vi "taskControllerExample.vi"() -> ()   [LabVIEW 2023]
uses:
  TaskController/TaskController.lvclass
  ITask/ITask.lvclass
panel:
  out "isRunning":bool
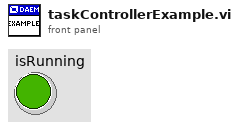
[diagram p1: front panel]
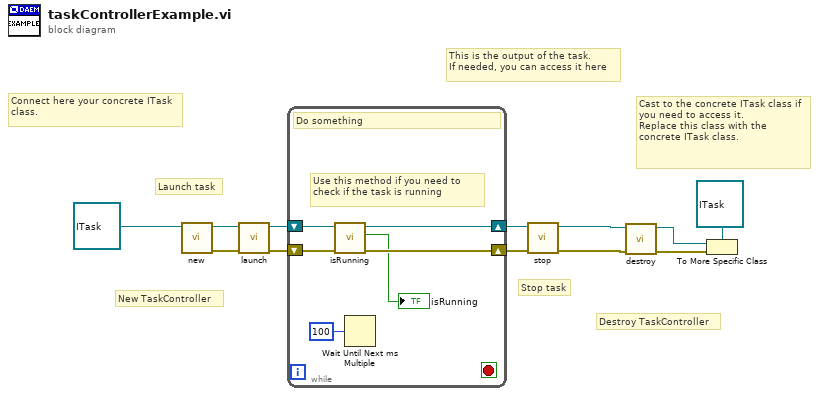
[diagram p0: block diagram]
diagram:
  # "Cast to the concrete ITask class if you need to access it.\nReplace this class with the concrete ITask class."
  # "This is the output of the task.\nIf needed, you can access it here"
  # "Connect here your concrete ITask class."
  # "Destroy TaskController"
  # "Stop task"
  # "Launch task"
  # "New TaskController"
  n1 = call "new.vi"("task"=refnum<class "ITask.lvclass"> refnum) -> ("error out"=w12:errorcluster, "TaskController out"=w11:refnum<class "TaskController.lvclass">)  [unwired: 9 in]
  n2 = call "launch.vi"("error in (no error)"=w12, "TaskController in"=w11) -> ("error out"=w10:errorcluster, "TaskController out"=w9:refnum<class "TaskController.lvclass">)  [unwired: 8 in]
  n3 = while {
    shift-right: [w16] -> w7
    shift-left: w9 -> [w17]
    shift-right: [w15] -> w8
    shift-left: w10 -> [w18]
    stop <- _ stop-if-true
    # "Use this method if you need to check if the task is running"
    # "Do something"
    n4 = call "isRunning.vi"("error in (no error)"=w18, "TaskController in"=w17) -> ("error out"=w15:errorcluster, "isRunning"=→"isRunning":bool, "TaskController out"=w16:refnum<class "TaskController.lvclass">)  [unwired: 7 in]
    n5 = Wait Until Next ms Multiple(millisecond multiple=u32 100 ("milliseconds to wait")) -> ()  [unwired: 1 out]
  }
  n6 = call "stop.vi"("error in (no error)"=w8, "TaskController in"=w7) -> ("error out"=w6:errorcluster, "TaskController out"=w5:refnum<class "TaskController.lvclass">)  [unwired: 8 in]
  n7 = call "destroy.vi"("error in (no error)"=w6, "TaskController in"=w5) -> ("error out"=w3:errorcluster, "taskResult"=w4:refnum<class "ITask.lvclass">)  [unwired: 7 in, 1 out]
  n8 = To More Specific Class(target class=refnum<class "ITask.lvclass"> refnum ("task"), reference=w4, error in=w3) -> ()  [unwired: 2 out]
